vi "Inputs.vi"() -> ()   [LabVIEW 2017]
panel:
  in  "Sharp_BL":dbl
  in  "Sharp_LB":dbl
  in  "Sharp_BR":dbl
  in  "Sharp_RB":dbl
  in  "Sharp_RF":dbl
  in  "Sharp_FR":dbl
  in  "Sharp_FL":dbl
  in  "Sharp_LF":dbl
  in  "Act_Vp":dbl
  in  "Act_Vy":dbl
  in  "Act_Vx":dbl
  in  "C1/Encoder":i32
  in  "C0/Encoder":i32
  in  "B/Encoder":i32
  in  "A/Encoder":i32
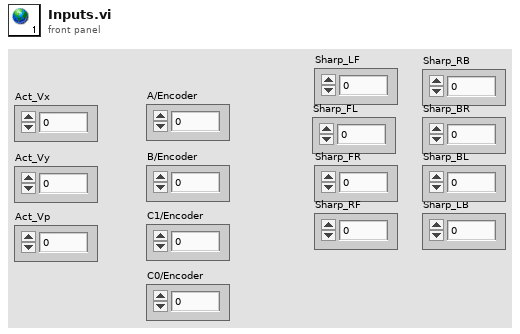
[diagram p1: front panel]
diagram:
